vi "UI-copper ring detection.vi"(8 "error in (no error)":errorcluster caption="错误输入（无错误）", 11 "名称或相对路径":string="Template Program") -> (0 "error in (no error) 2":errorcluster caption="错误输入（无错误）")   [LabVIEW 2017]
uses:
  Picture/SaveButtom.ctl
  <vilib>/vision/Measure.llb/Edge Options.ctl
  <vilib>/vision/Measure.llb/Edge Polarity.ctl
  Global System.vi
  <vilib>/Utility/xml.llb/Read From XML File(string).vi
  <vilib>/Utility/xml.llb/Write to XML File(string).vi
panel:
  in  "获取ROI(定位)":bool
  in  "采图按钮":bool
  in  "图像实时显示":bool
  in  "获取ROI(铜环)":bool
  out "Histogram (Histogram 1)":u32[][](array[numeric])
  out "添加的路径":path
  in  "刷新":bool
  in  "测试按钮":bool
  in  "保存按钮":bool
  in  "Main":enum32{"主参数", "圆环中心定位", "检测铜环参数 ", "测试效果"}(tab)
  in  "ParamsUI":T1={"IsNorImage"=TRUE, "Exposure Values"=100289, "ImagePath"=path "C:/Users/hedongpo/Desktop/514-hdp/Alignment Assemble System/Test Picture/B/3.bmp"} caption="参数界面" {"Exposure Values" scale=0.0..200000.0}
  in  "ParamsUI 圆环定位":T5={"圆环ROI设定"={"Center X"=1717, "Center Y"=1486, "Inner Radius"=327, "Outer Radius"=1645, "Start Angle"=0.0, "End Angle"=0.0}, "Options (定位)"={"Search  Direction"=0, "Edge Options"={"Edge Polarity"=0, "Kernel Size"=3, "Width"=3, "Minimum Edge Strength"=50.0, "Interpolation Type"=enum."Bilinear Fixed", "Data Processing Method"=enum."Average"}, "Show Search Area"=TRUE, "Show Search Lines"=TRUE, "Show Edges Found"=TRUE, "Show Result"=TRUE, "Search Area Color"=65280, "Search Lines Color"=255, "Edge Locations Color"=16776960, "Result Color"=16711680, "Overlay Group Name"=""}, "Circle Fit Options (定位)"={"Process"=enum."Get First Edge", "Step Size"=10, "Max Pixel Radius"=3}} caption="参数界面" {"Options (定位)"."Search  Direction" items=["Outside to Inside", "Inside to Outside"]; "Options (定位)"."Edge Options"."Edge Polarity" items=["All Edges", "Rising Edges", "Falling Edges"]; "Options (定位)"."Edge Options"."Minimum Edge Strength" format="%.2f"; "Options (定位)"."Edge Options"."Width" step=2; "Options (定位)"."Edge Options"."Kernel Size" step=2; "圆环ROI设定"."End Angle" min=-90.0 max=90.0 step=1.0 format="%.2f"; "圆环ROI设定"."Start Angle" min=-90.0 max=90.0 step=1.0 format="%.2f"; "圆环ROI设定"."Center X" scale=0.0..1024.0}
  in  "ParamsUI 内圆":cluster{"圆环ROI设定":T2, "黑像素个数判定阀值":dbl}={"圆环ROI设定"={"Center X"=1717, "Center Y"=1486, "Inner Radius"=327, "Outer Radius"=1645, "Start Angle"=0.0, "End Angle"=0.0}, "黑像素个数判定阀值"=0.0} caption="参数界面" {"圆环ROI设定"."End Angle" min=-90.0 max=90.0 step=1.0 format="%.2f"; "圆环ROI设定"."Start Angle" min=-90.0 max=90.0 step=1.0 format="%.2f"; "圆环ROI设定"."Center X" scale=0.0..1024.0}
  out "像素白个数":dbl
  out "像素黑个数":dbl
  out "原始图像":T6(plugin-control)
  out "Histogram 图标":u32[][](graph)
  out "路径输出":path
  in  "Vision Paramter Save Buttom":T7
  out "system time":string
  in  "取消按钮":bool
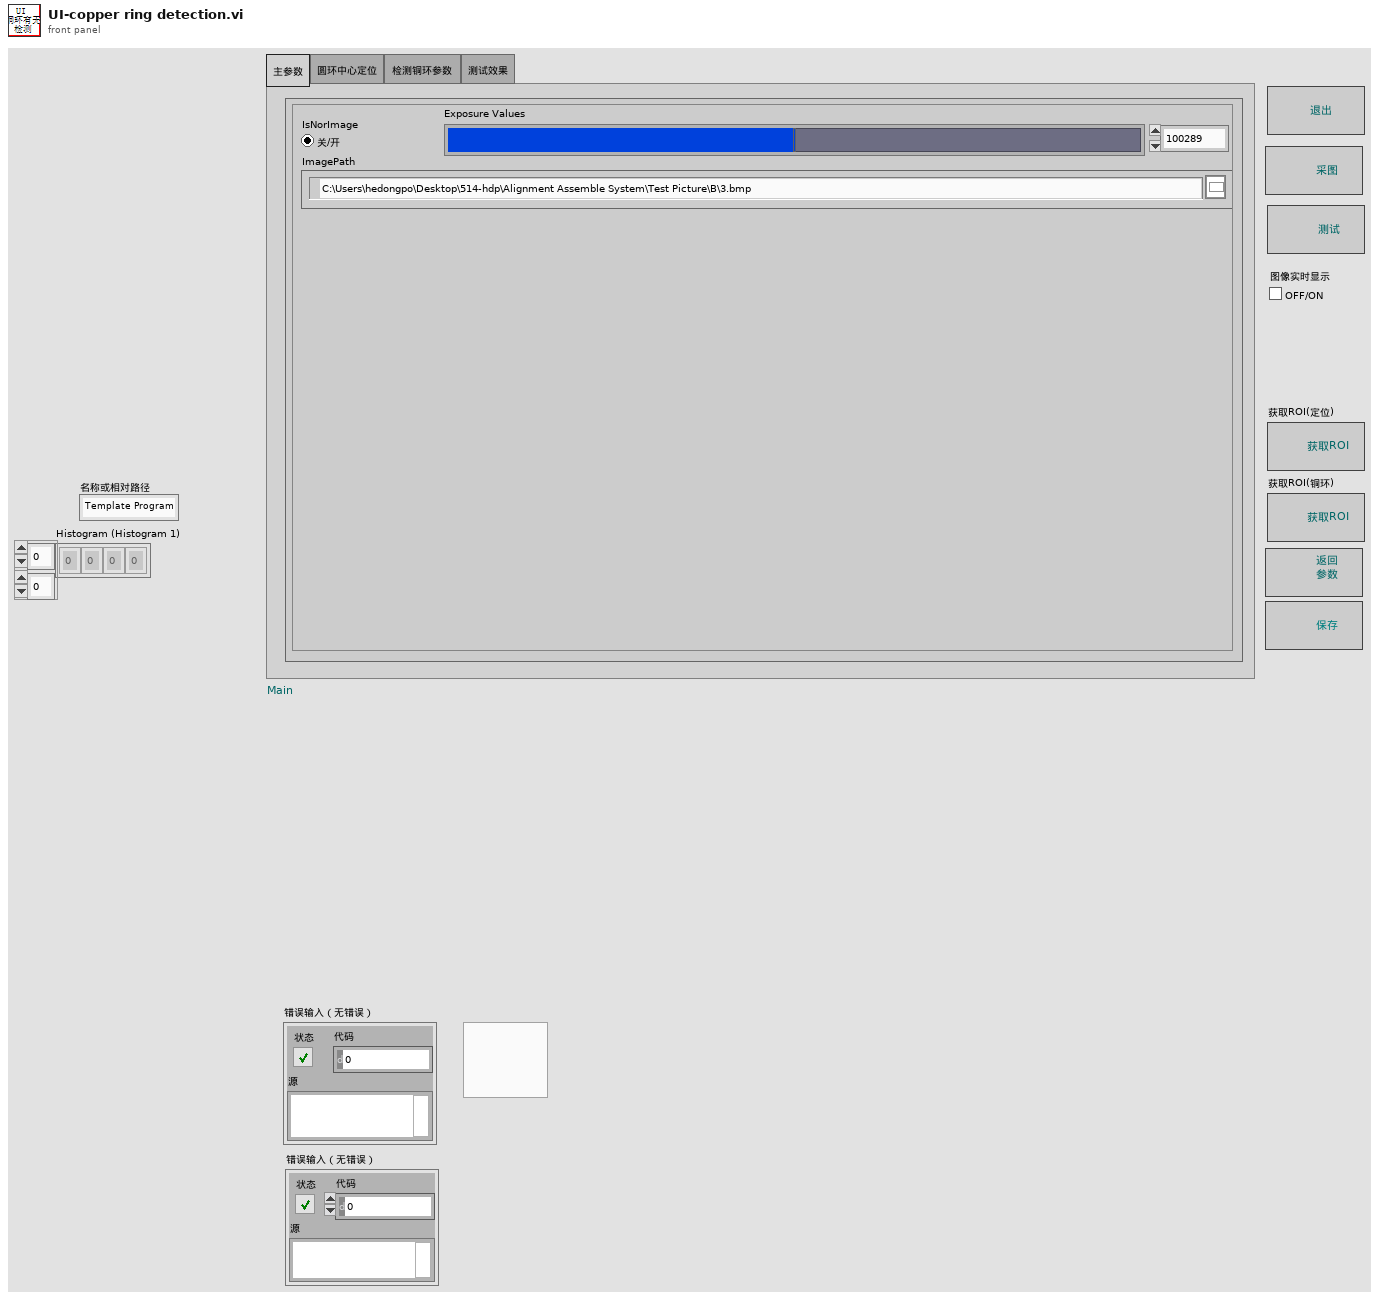
[diagram p1: front panel]
types:
  T1 = cluster{"IsNorImage":bool, "Exposure Values":u32, "ImagePath":path}
  T2 = typedef "IMAQ Circle" = cluster{"Center X":i32, "Center Y":i32, "Inner Radius":i32, "Outer Radius":i32, "Start Angle":dbl, "End Angle":dbl}
  T3 = typedef "Edge Options.ctl" = cluster{"Edge Polarity":T4, "Kernel Size":u32, "Width":u32, "Minimum Edge Strength":sgl, "Interpolation Type":enum32{"Zero Order", "Bilinear", "Quadratic", "Cubic", "Bilinear Fixed"}, "Data Processing Method":enum32{"Average", "Median"}}
  T4 = typedef "Edge Polarity.ctl" = u32
  T5 = cluster{"圆环ROI设定":T2, "Options (定位)":cluster{"Search  Direction":u32, "Edge Options":T3, "Show Search Area":bool, "Show Search Lines":bool, "Show Edges Found":bool, "Show Result":bool, "Search Area Color":u32, "Search Lines Color":u32, "Edge Locations Color":u32, "Result Color":u32, "Overlay Group Name":string}, "Circle Fit Options (定位)":cluster{"Process":enum16{"Get First Edge", "Get First + Last Edge", "Get All Edges", "Get Best Edge"}, "Step Size":i32, "Max Pixel Radius":i32}}
  T6 = typedef "IMAQ Image.ctl" = refnum<image>
  T7 = typedef "SaveButtom.ctl" = bool
  T8 = cluster{"扇区个数":string, "Fitted Circle (Find Circular Edge 1)":cluster{"Center (Pixels)":cluster{"X":sgl, "Y":sgl}, "Radius (Pixels)":dbl, "Center (Real-World)":cluster{"X":sgl, "Y":sgl}, "Radius (Real-World)":dbl, "Roundness (Real-World)":dbl, "Average Strength":dbl, "Average SNR (dB)":dbl}, "Range (Threshold 1)":cluster{"Lower value":sgl, "Upper value":sgl}, "Process (Edge Detector 1)":enum16{"Get First Edge", "Get First + Last Edge", "Get All Edges", "Get Best Edge"}, "Edge Options (Edge Detector 1)":cluster{"Edge Polarity":u32, "Kernel Size":u32, "Width":u32, "Minimum Edge Strength":sgl, "Interpolation Type":enum32{"Zero Order", "Bilinear", "Quadratic", "Cubic", "Bilinear Fixed"}, "Data Processing Method":enum32{"Average", "Median"}}}
  T9 = cluster{"index":i32, "this vi":refnum<vi>, "error out":errorcluster}
  T10 = cluster{"master data":string, "priority":u16, "secondary data":string[]}
  T11 = cluster{"case name":string[], "queue array":refnum<queue>[]}
  T12 = cluster{"Search  Direction":u32, "Edge Options":T3, "Show Search Area":bool, "Show Search Lines":bool, "Show Edges Found":bool, "Show Result":bool, "Search Area Color":u32, "Search Lines Color":u32, "Edge Locations Color":u32, "Result Color":u32, "Overlay Group Name":string}
  T13 = cluster{"Process":enum16{"Get First Edge", "Get First + Last Edge", "Get All Edges", "Get Best Edge"}, "Step Size":i32, "Max Pixel Radius":i32}
  T14 = typedef "ROI Descriptor" = cluster{"Global Rectangle":i32[], "Contours":cluster{"ID":enum32{"External", "Internal"}, "Type":u32, "Coordinates":i32[]}[]}
  T15 = cluster{"Center (Pixels)":cluster{"X":sgl, "Y":sgl}, "Radius (Pixels)":dbl, "Center (Real-World)":cluster{"X":sgl, "Y":sgl}, "Radius (Real-World)":dbl, "Roundness (Real-World)":dbl, "Average Strength":dbl, "Average SNR (dB)":dbl}
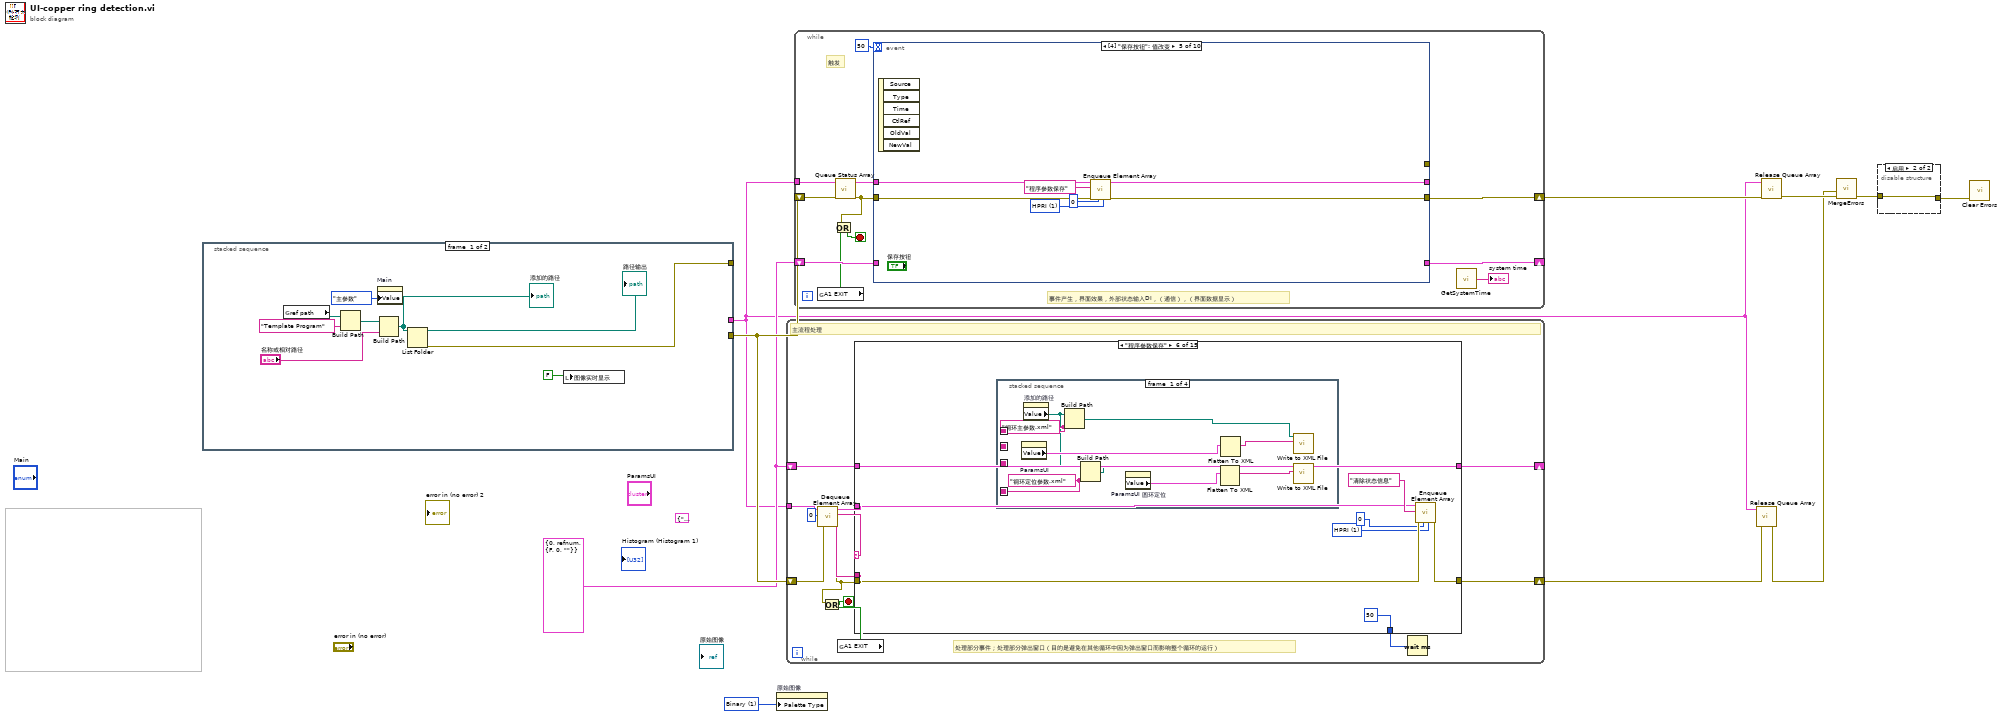
[diagram p0: block diagram]
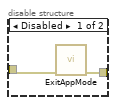
[diagram p2: hidden frame]
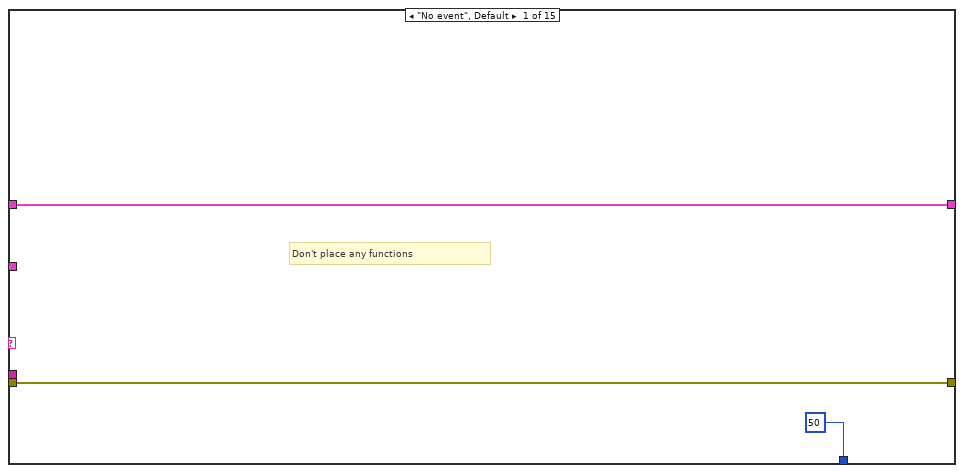
[diagram p3: hidden frame]
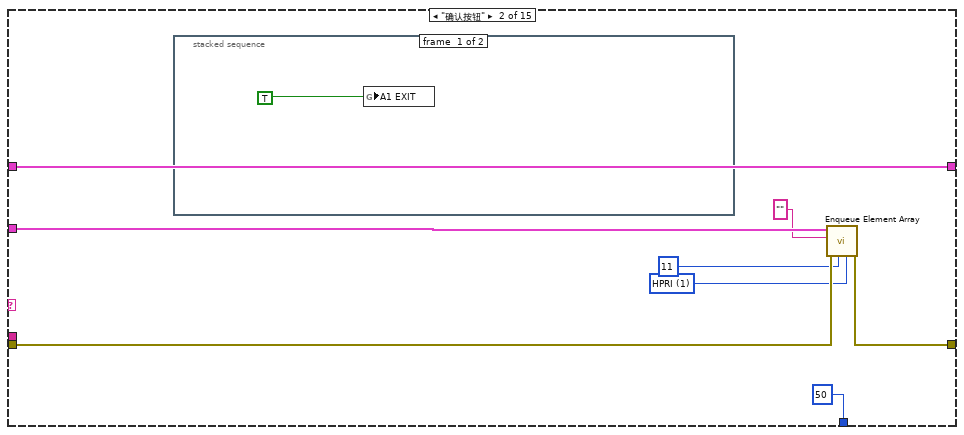
[diagram p4: hidden frame]
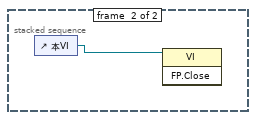
[diagram p5: hidden frame]
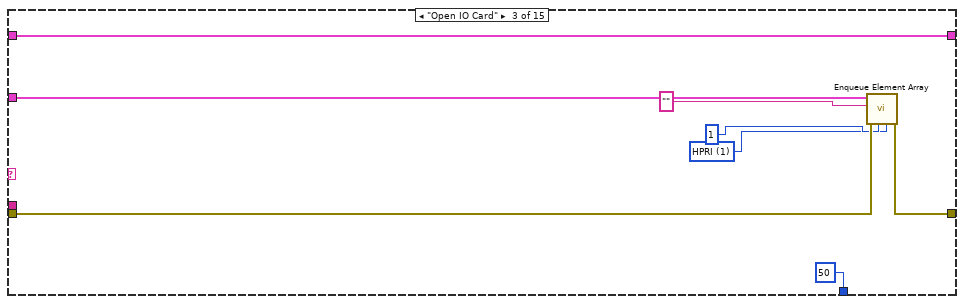
[diagram p6: hidden frame]
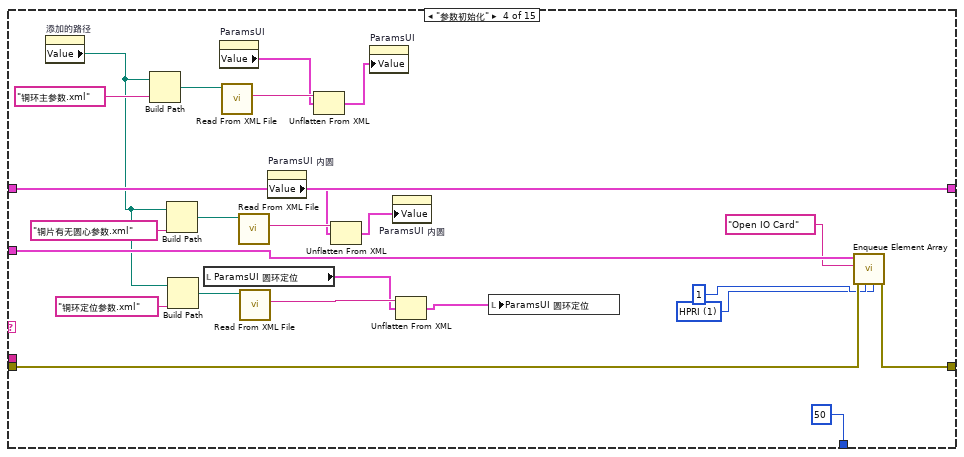
[diagram p7: hidden frame]
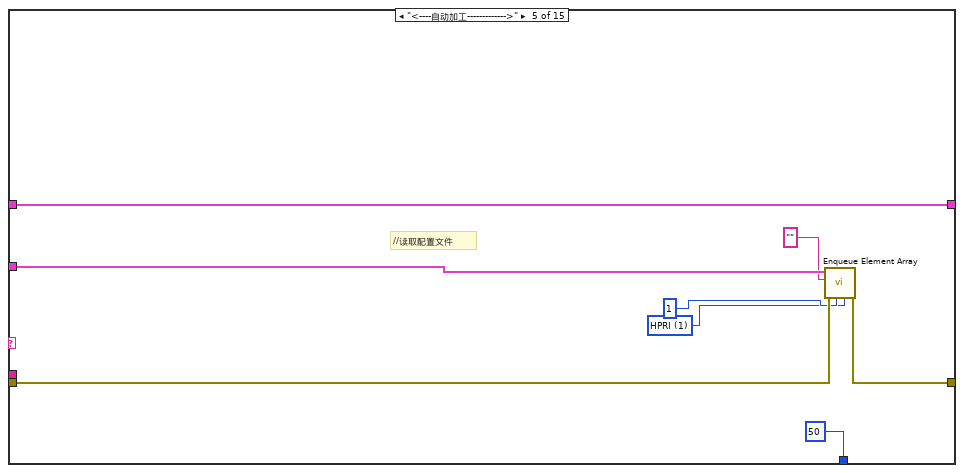
[diagram p8: hidden frame]
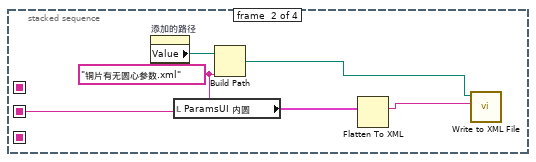
[diagram p9: hidden frame]
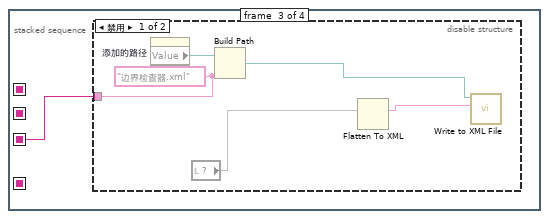
[diagram p10: hidden frame]
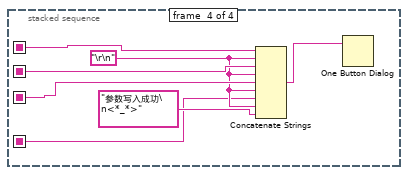
[diagram p12: hidden frame]
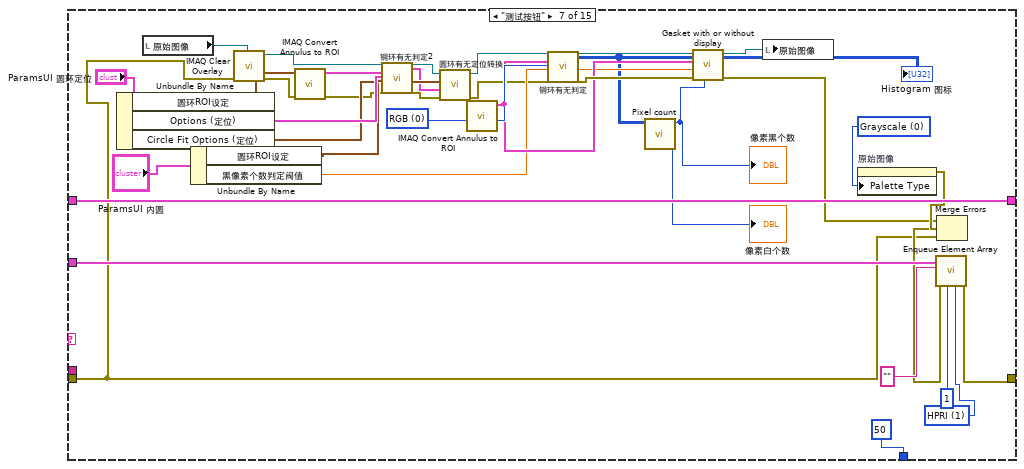
[diagram p13: hidden frame]
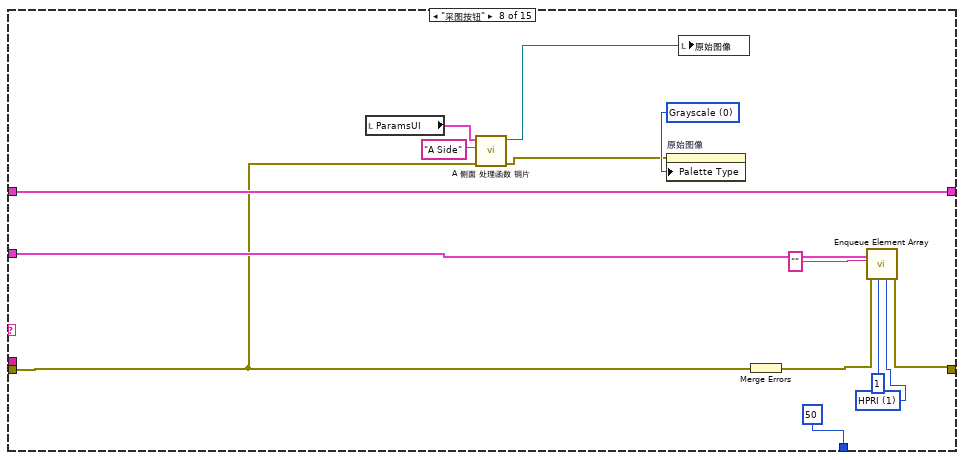
[diagram p14: hidden frame]
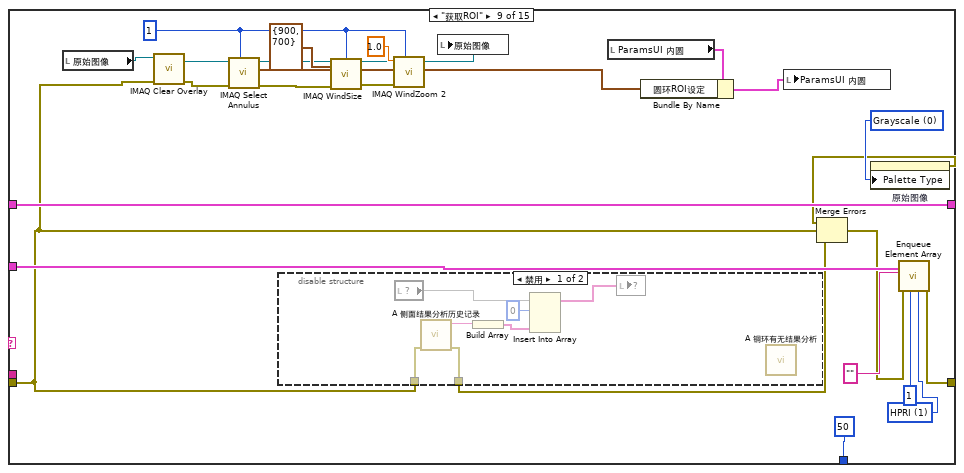
[diagram p15: hidden frame]
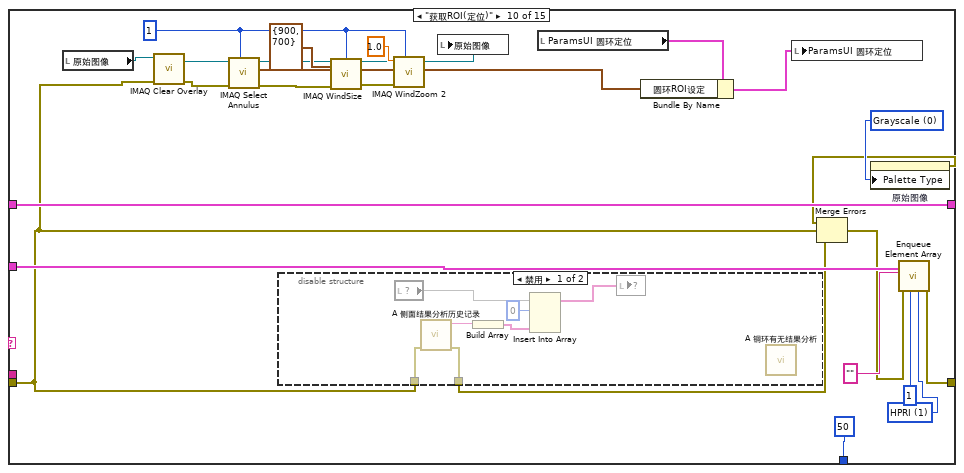
[diagram p17: hidden frame]
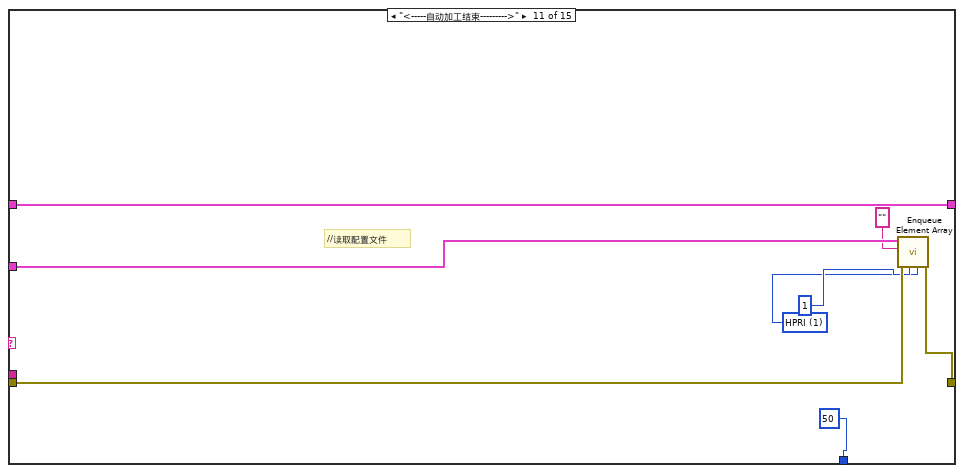
[diagram p19: hidden frame]
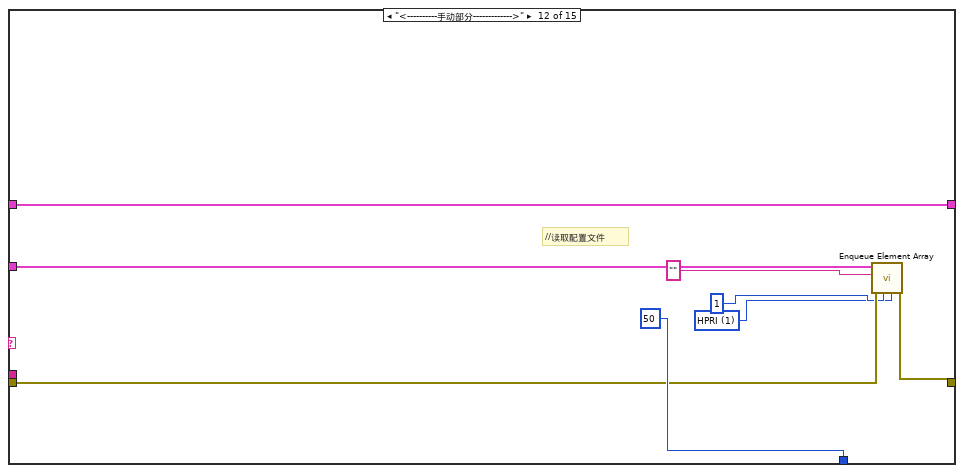
[diagram p20: hidden frame]
diagram:
  (unwired) T8 {"扇区个数"="1", "Fitted Circle (Find Circular Edge 1)"={"Center (Pixels)"={"X"=1736.0, "Y"=1501.0}, "Radius (Pixels)"=1442.0, "Center (Real-World)"={"X"=1736.0, "Y"=1501.0}, "Radius (Real-World)"=1442.0, "Roundness (Real-World)"=0.0, "Average Strength"=0.0, "Average SNR (dB)"=0.0}, "Range (Threshold 1)"={"Lower value"=65.0, "Upper value"=255.0}, "Process (Edge Detector 1)"=enum."Get All Edges", "Edge Options (Edge Detector 1)"={"Edge Polarity"=0, "Kernel Size"=9, "Width"=5, "Minimum Edge Strength"=27.0, "Interpolation Type"=enum."Bilinear", "Data Processing Method"=enum."Average"}} ("边界检查器参数")
  w1 = u32 1 items=["Grayscale", "Binary", "Gradient", "Rainbow", "Temperature", "User Defined", "Binary 16 Bit", "Gradient 16 Bit", "Rainbow 16 Bit", "Temperature 16 Bit", "User Defined 16 Bit"] ("Palette:Palette Type")
  w5 = T9 {"index"=0, "this vi"=refnum, "error out"={"status"=FALSE, "code"=0, "source"=""}} ("parameter buffer")
  n1 = stacked-sequence {
    tunnel: [w17 _] -> _
    tunnel: [_ w21] -> w6
    tunnel: [_ w20] -> w2
    frame #0 {
      n2 = global read "Global System.vi" "ref path"() -> (w15:path)
      n3 = Build Path(base path=w15, name or relative path="Template Program" ("名称或相对路径")) -> (appended path=w13:path)
      n4 = property on="Main" class="TabCtl (严格)"("Value"=enum32{"主参数", "圆环中心定位", "检测铜环参数 ", "测试效果"}."主参数" ("Main")) -> ()  [unwired: 2 in, 2 out]
      n5 = Build Path(base path=w13, name or relative path="名称或相对路径") -> (appended path=w19:path)
      "添加的路径" <- w19
      n6 = List Folder(path=w19) -> (path out=→"路径输出":path, error out=w17:errorcluster)  [unwired: 3 in, 2 out]
      n7 = local write "图像实时显示"(FALSE ("图像实时显示")) -> ()
    }
    frame #1 {
      w29 = string[] ["comm queue1", "data queue 11", "data queue 12", "data queue 13", "data queue 14"]  # queue name
      w30 = 4  # queue num
      w31 = T10 {"master data"="", "priority"=0, "secondary data"=[]}  # element data type
      n8 = call "Obtain Queue Array.vi"("queue name"=w29, "element data type"=w31, "queue num"=w30) -> ("error out"=w25:errorcluster, "queue out"=w26:T11)  [unwired: 2 in, 1 out]
      n9 = call "Enqueue Element Array.vi"("queue index"=0, "error in"=w25, "master data"="参数初始化", "queue in"=w26) -> ("error out"=w24:errorcluster, "queue out"=w23:T11)  [unwired: 6 in]
      n10 = disable-structure shown="启用" {
        disable-tunnel: w24 -> [w37 w38]
        disable-tunnel: w23 -> [w36 w39]
        disable-tunnel: "Loading Variable" ("master data") -> [w35 _]
        disable-tunnel: [w33 w38] -> w21
        disable-tunnel: [w32 w39] -> w20
        frame Disabled {
          n11 = call "Enqueue Element Array.vi"("queue index"=12, "error in"=w37, "master data"=w35, "queue in"=w36) -> ("error out"=w33:errorcluster, "queue out"=w32:T11)  [unwired: 6 in]
        }
        frame Enabled {
        }
      }
    }
  }
  n12 = property on="原始图像" class="ImageControl"("Palette Type"=w1) -> ()  [unwired: 2 in, 2 out]
  n13 = while {
    shift-right: [w52] -> w4
    shift-left: w6 -> [w43]
    shift-right: [w49] -> _
    shift-left: w5 -> [w50]
    tunnel: w2 -> [w45]
    stop <- w40 stop-if-true
    # "处理部分事件；处理部分弹出窗口（目的是避免在其他循环中因为弹出窗口而影响整个循环的运行）"
    # "主流程处理"
    n14 = call "Dequeue Element Array.vi"("queue in"=w45, "queue index"=0, "error in"=w43) -> ("queue out"=w48:T11, "master data"=w47:string, "secondary data"=w46:string[], "error out"=w42:errorcluster)  [unwired: 2 in, 1 out]
    n15 = global read "Global System.vi" "A1 EXIT"() -> (w41:bool)
    n16 = Or(x=w42, y=w41) -> (x .or. y?=w40:bool)
    n17 = case shown="\"程序参数保存\"" w47 {
      tunnel: w48 -> [_ w62 w72 w96 w104 w106 w177 w191 w215 w248 w265 w273 w281 w289 w295]
      tunnel: w42 -> [w54 w58 w68 w93 w100 w110 w143 w179 w195 w230 w261 w269 w277 w285 w292]
      tunnel: [w54 w61 w71 w95 w103 w112 w176 w190 w214 w247 w264 w272 w280 w288 w303] -> w52
      tunnel: [50 50 50 50 50 50 50 50 50 50 50 50 50 50 50] -> w51
      tunnel: w50 -> [w55 w59 w69 w90 w101 w107 w172 w186 w210 w243 w262 w270 w278 w286 w301]
      tunnel: [w55 w59 w69 w90 w101 w107 w172 w186 w210 w243 w262 w270 w278 w286 w301] -> w49
      tunnel: w46 -> [_ _ _ _ _ _ _ _ _ _ _ _ _ _ _]
      frame "No event", Default {
        # "Don't place any functions"
      }
      frame "确认按钮" {
        w56 = u16 1 items=["HPRI"=1, "LPRI"=0] ("priority")
        n18 = stacked-sequence {
          frame #0 {
            n19 = global write "Global System.vi" "A1 EXIT"(TRUE ("EXIT")) -> ()
          }
          frame #1 {
            n20 = control-ref of="本VI"() -> (w65:refnum<vi>)
            n21 = invoke class="VI" method="FP.Close"(reference=w65) -> ()  [unwired: 2 in, 3 out]
          }
        }
        n22 = call "Enqueue Element Array.vi"("priority"=w56, "queue index"=11, "error in"=w58, "master data"="" ("Element 1"), "queue in"=w62) -> ("error out"=w61:errorcluster)  [unwired: 5 in, 1 out]
      }
      frame "Open IO Card" {
        w66 = u16 1 items=["HPRI"=1, "LPRI"=0] ("priority")
        n23 = call "Enqueue Element Array.vi"("priority"=w66, "queue index"=1, "error in"=w68, "master data"="" ("Element 1"), "queue in"=w72) -> ("error out"=w71:errorcluster)  [unwired: 5 in, 1 out]
      }
      frame "参数初始化" {
        w91 = u16 1 items=["HPRI"=1, "LPRI"=0] ("priority")
        n24 = property on="添加的路径" class="Path"() -> ("Value"=w76:path)  [unwired: 2 in, 2 out]
        n25 = Build Path(base path=w76, name or relative path="铜环主参数.xml" ("名称或相对路径")) -> (appended path=w88:path)
        n26 = Build Path(base path=w76, name or relative path="铜片有无圆心参数.xml" ("名称或相对路径")) -> (appended path=w83:path)
        n27 = Build Path(base path=w76, name or relative path="铜环定位参数.xml" ("名称或相对路径")) -> (appended path=w78:path)
        n28 = local read "ParamsUI 圆环定位"() -> (w74:T5)
        n29 = property on="ParamsUI" class="Clust (严格)"() -> ("Value"=w86:T1)  [unwired: 2 in, 2 out]
        n30 = call-poly <vilib>:"Read From XML File.vi"("XML File Path"=w88) -> ("XML Elements"=w87:string)  [unwired: 8 in, 2 out]
        n31 = call-poly <vilib>:"Read From XML File.vi"("XML File Path"=w83) -> ("XML Elements"=w84:string)  [unwired: 8 in, 2 out]
        n32 = call-poly <vilib>:"Read From XML File.vi"("XML File Path"=w78) -> ("XML Elements"=w77:string)  [unwired: 8 in, 2 out]
        n33 = property on="ParamsUI 内圆" class="Clust (严格)"() -> ("Value"=w81:cluster{"圆环ROI设定":T2, "黑像素个数判定阀值":dbl})  [unwired: 2 in, 2 out]
        n34 = Unflatten From XML(xml string=w87, type=w86) -> (value=w85:T1)  [unwired: 1 in, 1 out]
        n35 = Unflatten From XML(xml string=w84, type=w81) -> (value=w80:cluster{"圆环ROI设定":T2, "黑像素个数判定阀值":dbl})  [unwired: 1 in, 1 out]
        n36 = property on="ParamsUI" class="Clust (严格)"("Value"=w85) -> ()  [unwired: 2 in, 2 out]
        n37 = property on="ParamsUI 内圆" class="Clust (严格)"("Value"=w80) -> ()  [unwired: 2 in, 2 out]
        n38 = Unflatten From XML(xml string=w77, type=w74) -> (value=w75:T5)  [unwired: 1 in, 1 out]
        n39 = local write "ParamsUI 圆环定位"(w75) -> ()
        n40 = call "Enqueue Element Array.vi"("priority"=w91, "queue index"=1, "error in"=w93, "master data"="Open IO Card" ("Element 1"), "queue in"=w96) -> ("error out"=w95:errorcluster)  [unwired: 5 in, 1 out]
      }
      frame "<----自动加工------------->" {
        w98 = u16 1 items=["HPRI"=1, "LPRI"=0] ("priority")
        # "//读取配置文件"
        n41 = call "Enqueue Element Array.vi"("priority"=w98, "queue index"=1, "error in"=w100, "master data"="" ("Element 1"), "queue in"=w104) -> ("error out"=w103:errorcluster)  [unwired: 5 in, 1 out]
      }
      frame "程序参数保存" {
        w108 = u16 1 items=["HPRI"=1, "LPRI"=0] ("priority")
        n42 = stacked-sequence {
          seq-local: [w119 _ _ _] -> [_ _ _ w139]
          seq-local: [_ w123 _ _] -> [_ _ _ w137]
          seq-local: [_ _ w128 _] -> [_ _ _ w136]
          seq-local: [w114 _ _ _] -> [_ _ _ w134]
          frame #0 {
            w114 = "铜环定位参数.xml" ("名称或相对路径")
            w119 = "铜环主参数.xml" ("名称或相对路径")
            n43 = property on="ParamsUI" class="Clust (严格)"() -> ("Value"=w122:T1)  [unwired: 2 in, 2 out]
            n44 = property on="添加的路径" class="Path"() -> ("Value"=w118:path)  [unwired: 2 in, 2 out]
            n45 = Build Path(base path=w118, name or relative path=w119) -> (appended path=w120:path)
            n46 = Build Path(base path=w118, name or relative path=w114) -> (appended path=w117:path)
            n47 = property on="ParamsUI 圆环定位" class="Clust (严格)"() -> ("Value"=w116:T5)  [unwired: 2 in, 2 out]
            n48 = Flatten To XML(anything=w116) -> (xml string=w115:string)
            n49 = Flatten To XML(anything=w122) -> (xml string=w121:string)
            n50 = call-poly <vilib>:"Write to XML File.vi"("XML Input"=w121, "XML File Path"=w120) -> ()  [unwired: 7 in, 3 out]
            n51 = call-poly <vilib>:"Write to XML File.vi"("XML Input"=w115, "XML File Path"=w117) -> ()  [unwired: 7 in, 3 out]
          }
          frame #1 {
            w123 = "铜片有无圆心参数.xml" ("名称或相对路径")
            n52 = property on="添加的路径" class="Path"() -> ("Value"=w127:path)  [unwired: 2 in, 2 out]
            n53 = local read "ParamsUI 内圆"() -> (w124:cluster{"圆环ROI设定":T2, "黑像素个数判定阀值":dbl})
            n54 = Build Path(base path=w127, name or relative path=w123) -> (appended path=w125:path)
            n55 = Flatten To XML(anything=w124) -> (xml string=w126:string)
            n56 = call-poly <vilib>:"Write to XML File.vi"("XML Input"=w126, "XML File Path"=w125) -> ()  [unwired: 7 in, 3 out]
          }
          frame #2 {
            n57 = disable-structure shown="禁用" {
              disable-tunnel: [w130 _] -> w128
              frame Disabled {
                w130 = "边界检查器.xml" ("名称或相对路径")
                n58 = property on="添加的路径" class="Path"() -> ("Value"=w133:path)  [unwired: 2 in, 2 out]
                n59 = local read item#-1() -> (w129)
                n60 = Build Path(base path=w133, name or relative path=w130) -> (appended path=w131:path)
                n61 = Flatten To XML(anything=w129) -> (xml string=w132:string)
                n62 = call-poly <vilib>:"Write to XML File.vi"("XML Input"=w132, "XML File Path"=w131) -> ()  [unwired: 7 in, 3 out]
              }
              frame Enabled {
              }
            }
          }
          frame #3 {
            w135 = "\r\n"
            n63 = Concatenate Strings(w139, w135, w137, w135, w136, w135, w134, w135, "参数写入成功\n<*_*>" ("消息")) -> (w138:string)
            n64 = One Button Dialog(message=w138) -> ()  [unwired: 1 in, 1 out]
          }
        }
        n65 = call "Enqueue Element Array.vi"("priority"=w108, "queue index"=0, "error in"=w110, "master data"="清除状态信息" ("Element 1"), "queue in"=w106) -> ("error out"=w112:errorcluster)  [unwired: 5 in, 1 out]
      }
      frame "测试按钮" {
        w167 = u16 0 items=["RGB", "HSL", "HSV", "HSI"] ("Color Mode (Histogram 1)")
        w171 = u32 0 items=["Grayscale", "Binary", "Gradient", "Rainbow", "Temperature", "User Defined", "Binary 16 Bit", "Gradient 16 Bit", "Rainbow 16 Bit", "Temperature 16 Bit", "User Defined 16 Bit"] ("Palette:Palette Type")
        w173 = u16 1 items=["HPRI"=1, "LPRI"=0] ("priority")
        n66 = Unbundle By Name("ParamsUI 圆环定位") -> ("圆环ROI设定"=w156:T2, "Options (定位)"=w154:T12, "Circle Fit Options (定位)"=w153:T13)
        n67 = local read "原始图像"() -> (w158:T6)
        n68 = Unbundle By Name("ParamsUI 内圆") -> ("圆环ROI设定"=w152:T2, "黑像素个数判定阀值"=w160:dbl)
        n69 = call "IMAQ Clear Overlay"("error in (no error)"=w143, "Image"=w158) -> ("error out"=w144:errorcluster, "Image Out"=w145:T6)  [unwired: 8 in]
        n70 = call "IMAQ Convert Annulus to ROI"("error in (no error)"=w144, "Annulus"=w156) -> ("error out"=w142:errorcluster, "ROI Descriptor"=w155:T14)  [unwired: 7 in]
        n71 = call "铜环有无判定2"("Image In"=w145, "ROI Descriptor (Find Circular Edge 1)"=w155, "Options (Find Circular Edge 1)"=w154, "Circle Fit Options (Find Circular Edge 1)"=w153, "error in"=w142) -> ("Image Out"=w149:T6, "Fitted Circle (Find Circular Edge 1)"=w150:T15, "error out"=w147:errorcluster)  [unwired: 20 in]
        n72 = call "圆环有无定位转换.vi"("error in (no error)"=w147, "Fitted Circle (定位)"=w150, "圆环ROI设定 in"=w152, "Image in"=w149) -> ("error out"=w146:errorcluster, "圆环ROI设定 out"=w151:T2, "Image out"=w148:T6)  [unwired: 4 in, 1 out]
        n73 = call "IMAQ Convert Annulus to ROI"("Annulus"=w151) -> ("ROI Descriptor"=w162:T14)  [unwired: 8 in, 1 out]
        n74 = call "铜环有无判定"("Image In"=w148, "ROI Descriptor (Histogram 1)"=w162, "Color Mode (Histogram 1)"=w167, "error in"=w146) -> ("Image Out"=w166:T6, "Histogram (Histogram 1)"=w141:u32[][], "error out"=w164:errorcluster)  [unwired: 20 in, 1 out]
        "Histogram 图标" <- w141
        n75 = call "Pixel count.vi"("Histogram 图标"=w141) -> ("像素白个数"=→"像素白个数":u32, "像素黑个数"=w159:u32)  [unwired: 9 in]
        "像素黑个数" <- w159
        n76 = call "Gasket with or without display.vi"("黑像个数"=w159, "error in (no error)"=w164, "黑像素阀值判定个数"=w160, "ROI Descriptor"=w162, "原始图像 IN"=w166) -> ("error out"=w163:errorcluster, "原始图像 OUT"=w165:T6)  [unwired: 3 in, 2 out]
        n77 = local write "原始图像"(w165) -> ()
        n78 = property on="原始图像" class="ImageControl"("Palette Type"=w171) -> (error out=w170:errorcluster)  [unwired: 2 in, 1 out]
        n79 = Merge Errors(w163, w170, w143) -> (w169:errorcluster)
        n80 = call "Enqueue Element Array.vi"("priority"=w173, "queue index"=1, "error in"=w169, "master data"="" ("Element 1"), "queue in"=w177) -> ("error out"=w176:errorcluster)  [unwired: 5 in, 1 out]
      }
      frame "采图按钮" {
        w184 = u32 0 items=["Grayscale", "Binary", "Gradient", "Rainbow", "Temperature", "User Defined", "Binary 16 Bit", "Gradient 16 Bit", "Rainbow 16 Bit", "Temperature 16 Bit", "User Defined 16 Bit"] ("Palette:Palette Type")
        w187 = u16 1 items=["HPRI"=1, "LPRI"=0] ("priority")
        n81 = local read "ParamsUI"() -> (w183:T1)
        n82 = call "A 侧面 处理函数 铜片.vi"("error in (no error)"=w179, "Image Name"="A Side", "ParamsUI"=w183) -> ("error out"=w180:errorcluster, "Image out"=w181:T6)  [unwired: 5 in, 2 out]
        n83 = property on="原始图像" class="ImageControl"(error in=w180, "Palette Type"=w184) -> ()  [unwired: 1 in, 2 out]
        n84 = local write "原始图像"(w181) -> ()
        n85 = Merge Errors(w179) -> (w182:errorcluster)
        n86 = call "Enqueue Element Array.vi"("priority"=w187, "queue index"=1, "error in"=w182, "master data"="" ("Element 1"), "queue in"=w191) -> ("error out"=w190:errorcluster)  [unwired: 5 in, 1 out]
      }
      frame "获取ROI" {
        w203 = 1 ("Window Number (0...15)")
        w209 = u32 0 items=["Grayscale", "Binary", "Gradient", "Rainbow", "Temperature", "User Defined", "Binary 16 Bit", "Gradient 16 Bit", "Rainbow 16 Bit", "Temperature 16 Bit", "User Defined 16 Bit"] ("Palette:Palette Type")
        w211 = u16 1 items=["HPRI"=1, "LPRI"=0] ("priority")
        n87 = local read "原始图像"() -> (w196:T6)
        n88 = call "IMAQ Clear Overlay"("error in (no error)"=w195, "Image"=w196) -> ("error out"=w194:errorcluster, "Image Out"=w193:T6)  [unwired: 8 in]
        n89 = call "IMAQ Select Annulus"("Window Number (0...15)"=w203, "error in (no error)"=w194, "Image In"=w193) -> ("error out"=w205:errorcluster, "Annulus"=w198:T2, "Image Out (duplicate)"=w200:T6)  [unwired: 5 in, 1 out]
        n90 = disable-structure shown="禁用" {
          disable-tunnel: w195 -> [w220 _]
          disable-tunnel: [w219 _] -> w206
          frame Disabled {
            n91 = local read item#-1() -> (w218)
            n92 = call "A 侧面结果分析历史记录.vi"("错误输入（无错误）"=w220) -> ("错误输出"=w219:errorcluster, "F-格式字符串"=w223:string, "Tbl引用句柄"=w221:refnum<vi>)  [unwired: 8 in]
            n93 = Build Array(w223) -> (w222:string[])
            n94 = Insert Into Array(array=w218, index (row)=0 ("索引 (行)"), new element=w222) -> (w217:string[])  [unwired: 1 in]
            n95 = local write item#-1(w217) -> ()
            n96 = call "A 铜环有无结果分析.vi"() -> ("Tbl引用句柄"=w225:refnum<vi>)  [unwired: 11 in]
          }
          frame Enabled {
          }
        }
        n97 = call "IMAQ WindSize"("error in (no error)"=w205, "Width & Height"=cluster{"Width":i32, "Height":i32} {"Width"=900, "Height"=700}, "Window Number"=w203) -> ("error out"=w202:errorcluster)  [unwired: 3 in, 2 out]
        n98 = call "IMAQ WindZoom 2"("Window Number (0...15)"=w203, "error in (no error)"=w202, "Zoom Factor"=sgl 1.0) -> ()  [unwired: 5 in, 4 out]
        n99 = local write "原始图像"(w200) -> ()
        n100 = local read "ParamsUI 内圆"() -> (w199:cluster{"圆环ROI设定":T2, "黑像素个数判定阀值":dbl})
        n101 = Bundle By Name(cluster=w199, "圆环ROI设定"=w198) -> (w197:cluster{"圆环ROI设定":T2, "黑像素个数判定阀值":dbl})
        n102 = local write "ParamsUI 内圆"(w197) -> ()
        n103 = property on="原始图像" class="ImageControl"("Palette Type"=w209) -> (error out=w208:errorcluster)  [unwired: 2 in, 1 out]
        n104 = Merge Errors(w208, w195, w206) -> (w207:errorcluster)
        n105 = call "Enqueue Element Array.vi"("priority"=w211, "queue index"=1, "error in"=w207, "master data"="" ("Element 1"), "queue in"=w215) -> ("error out"=w214:errorcluster)  [unwired: 5 in, 1 out]
      }
      frame "获取ROI(定位)" {
        w236 = 1 ("Window Number (0...15)")
        w242 = u32 0 items=["Grayscale", "Binary", "Gradient", "Rainbow", "Temperature", "User Defined", "Binary 16 Bit", "Gradient 16 Bit", "Rainbow 16 Bit", "Temperature 16 Bit", "User Defined 16 Bit"] ("Palette:Palette Type")
        w244 = u16 1 items=["HPRI"=1, "LPRI"=0] ("priority")
        n106 = local read "原始图像"() -> (w231:T6)
        n107 = call "IMAQ Clear Overlay"("error in (no error)"=w230, "Image"=w231) -> ("error out"=w229:errorcluster, "Image Out"=w228:T6)  [unwired: 8 in]
        n108 = call "IMAQ Select Annulus"("Window Number (0...15)"=w236, "error in (no error)"=w229, "Image In"=w228) -> ("error out"=w238:errorcluster, "Annulus"=w232:T2, "Image Out (duplicate)"=w233:T6)  [unwired: 5 in, 1 out]
        n109 = disable-structure shown="禁用" {
          disable-tunnel: w230 -> [w253 _]
          disable-tunnel: [w252 _] -> w239
          frame Disabled {
            n110 = local read item#-1() -> (w251)
            n111 = call "A 侧面结果分析历史记录.vi"("错误输入（无错误）"=w253) -> ("错误输出"=w252:errorcluster, "F-格式字符串"=w256:string, "Tbl引用句柄"=w254:refnum<vi>)  [unwired: 8 in]
            n112 = Build Array(w256) -> (w255:string[])
            n113 = Insert Into Array(array=w251, index (row)=0 ("索引 (行)"), new element=w255) -> (w250:string[])  [unwired: 1 in]
            n114 = local write item#-1(w250) -> ()
            n115 = call "A 铜环有无结果分析.vi"() -> ("Tbl引用句柄"=w258:refnum<vi>)  [unwired: 11 in]
          }
          frame Enabled {
          }
        }
        n116 = call "IMAQ WindSize"("error in (no error)"=w238, "Width & Height"=cluster{"Width":i32, "Height":i32} {"Width"=900, "Height"=700}, "Window Number"=w236) -> ("error out"=w235:errorcluster)  [unwired: 3 in, 2 out]
        n117 = call "IMAQ WindZoom 2"("Window Number (0...15)"=w236, "error in (no error)"=w235, "Zoom Factor"=sgl 1.0) -> ()  [unwired: 5 in, 4 out]
        n118 = local write "原始图像"(w233) -> ()
        n119 = local read "ParamsUI 圆环定位"() -> (w227:T5)
        n120 = Bundle By Name(cluster=w227, "圆环ROI设定"=w232) -> (w226:T5)
        n121 = local write "ParamsUI 圆环定位"(w226) -> ()
        n122 = property on="原始图像" class="ImageControl"("Palette Type"=w242) -> (error out=w241:errorcluster)  [unwired: 2 in, 1 out]
        n123 = Merge Errors(w241, w230, w239) -> (w240:errorcluster)
        n124 = call "Enqueue Element Array.vi"("priority"=w244, "queue index"=1, "error in"=w240, "master data"="" ("Element 1"), "queue in"=w248) -> ("error out"=w247:errorcluster)  [unwired: 5 in, 1 out]
      }
      frame "<-----自动加工结束--------->" {
        w259 = u16 1 items=["HPRI"=1, "LPRI"=0] ("priority")
        # "//读取配置文件"
        n125 = call "Enqueue Element Array.vi"("priority"=w259, "queue index"=1, "error in"=w261, "master data"="" ("Element 1"), "queue in"=w265) -> ("error out"=w264:errorcluster)  [unwired: 5 in, 1 out]
      }
      frame "<----------手动部分------------->" {
        w267 = u16 1 items=["HPRI"=1, "LPRI"=0] ("priority")
        # "//读取配置文件"
        n126 = call "Enqueue Element Array.vi"("priority"=w267, "queue index"=1, "error in"=w269, "master data"="" ("Element 1"), "queue in"=w273) -> ("error out"=w272:errorcluster)  [unwired: 5 in, 1 out]
      }
      frame "参数设置保存" {
        w275 = u16 1 items=["HPRI"=1, "LPRI"=0] ("priority")
        n127 = call "Enqueue Element Array.vi"("priority"=w275, "queue index"=1, "error in"=w277, "master data"="" ("Element 1"), "queue in"=w281) -> ("error out"=w280:errorcluster)  [unwired: 5 in, 1 out]
      }
      frame "<--------------手动结束---------------->" {
        w283 = u16 1 items=["HPRI"=1, "LPRI"=0] ("priority")
        # "//读取配置文件"
        n128 = call "Enqueue Element Array.vi"("priority"=w283, "queue index"=1, "error in"=w285, "master data"="" ("Element 1"), "queue in"=w289) -> ("error out"=w288:errorcluster)  [unwired: 5 in, 1 out]
      }
      frame "*Emergency alarm" {
        w298 = u16 1 items=["HPRI"=1, "LPRI"=0] ("priority")
        w299 = u16 1 items=["HPRI"=1, "LPRI"=0] ("priority")
        # "发出处理急停信号的命令"
        # "发出处理急停信号的命令"
        n129 = call "Enqueue Element Array.vi"("priority"=w298, "queue index"=0, "error in"=w292, "master data"="" ("Element 1"), "queue in"=w295) -> ("error out"=w293:errorcluster, "queue out"=w294:T11)  [unwired: 5 in]
        n130 = call "SetTestInfoIndex.vi"("test info index"=13) -> ()
        n131 = call "Enqueue Element Array.vi"("priority"=w299, "queue index"=1, "error in"=w293, "master data"="" ("Element 1"), "queue in"=w294) -> ("error out"=w303:errorcluster)  [unwired: 5 in, 1 out]
      }
    }
    n132 = Wait (ms)(milliseconds to wait=w51) -> ()  [unwired: 1 out]
  }
  n133 = while {
    shift-right: [w308] -> w7
    shift-left: w6 -> [w312]
    shift-right: [w310] -> _
    shift-left: w5 -> [w311]
    tunnel: w2 -> [w314]
    stop <- w305 stop-if-true
    # "触发"
    # "事件产生，界面效果，外部状态输入DI，（通信），（界面数据显示）"
    n134 = global read "Global System.vi" "A1 EXIT"() -> (w306:bool)
    n135 = call "Queue Status Array.vi"("error in (no error)"=w312, "queue in"=w314) -> ("error out"=w307:errorcluster, "queue out"=w309:T11)  [unwired: 4 in]
    n136 = Or(x=w307, y=w306) -> (x .or. y?=w305:bool)
    n137 = event shown="[4] \"保存按钮\": 值改变" {
      selector: _ -> [_ _ _ _ _ _ _ _ _ _]
      dyn-events: _ -> [_ _ _ _ _ _ _ _ _ _]
      timeout: 50 -> [_ _ _ _ _ _ _ _ _ _]
      tunnel: w311 -> [w320 w334 _ _ _ _ _ _ _ _]
      tunnel: [w320 w334 _ _ _ _ _ _ _ _] -> w310
      tunnel: [errorcluster {"status"=FALSE, "code"=0, "source"=""} ("error out") _ _ _ _ _ _ _ _ _] -> _
      tunnel: w309 -> [w318 w333 w339 w346 w353 w361 w369 w377 w385 w393]
      tunnel: w307 -> [w316 w332 w338 w345 w352 w360 w368 w376 w384 w392]
      tunnel: [w316 w331 w336 w343 w350 w358 w366 w374 w382 w390] -> w308
      tunnel: [w318 w330 w337 w344 w351 w359 w367 w375 w383 w391] -> _
      event Timeout {
        # "不要在事件结构里面放入\"弹出窗口\"这样的VI保证该循环畅通无阻。"
        n138 = event-data() -> ()  [unwired: 1 in, 1 out]
        n139 = case shown="真" "图像实时显示" {
          tunnel: w316 -> [_ w321]
          frame False {
          }
          frame True {
            w323 = u32 0 items=["Grayscale", "Binary", "Gradient", "Rainbow", "Temperature", "User Defined", "Binary 16 Bit", "Gradient 16 Bit", "Rainbow 16 Bit", "Temperature 16 Bit", "User Defined 16 Bit"] ("Palette:Palette Type")
            n140 = local read "ParamsUI"() -> (w326:T1)
            n141 = call "Get aperture images CCD2.vi"("error in (no error)"=w321, "Image Name"="A Side", "ParamsUI"=w326) -> ("error out"=w322:errorcluster, "Image out"=w324:T6)  [unwired: 5 in, 2 out]
            n142 = property on="原始图像" class="ImageControl"(error in=w322, "Palette Type"=w323) -> ()  [unwired: 1 in, 2 out]
            n143 = local write "原始图像"(w324) -> ()
          }
        }
      }
      event Panel Close? {
        w328 = u16 1 items=["HPRI"=1, "LPRI"=0] ("priority")
        n144 = event-data() -> ()  [unwired: 1 in, 4 out]
        n145 = call "Enqueue Element Array.vi"("priority"=w328, "queue index"=0, "error in"=w332, "master data"="*Exit application", "queue in"=w333) -> ("error out"=w331:errorcluster, "queue out"=w330:T11)  [unwired: 5 in]
        n146 = event-data("Discard?"=TRUE) -> ()  [unwired: 1 in, 1 out]
      }
      event Value Change {
        w341 = u16 1 items=["HPRI"=1, "LPRI"=0] ("priority")
        n147 = event-data() -> ()  [unwired: 1 in, 6 out]
        n148 = call "Enqueue Element Array.vi"("priority"=w341, "queue index"=0, "error in"=w338, "master data"="Vision Paramter Save", "queue in"=w339) -> ("error out"=w336:errorcluster, "queue out"=w337:T11)  [unwired: 5 in]
      }
      event "取消按钮": Value Change {
        w348 = u16 1 items=["HPRI"=1, "LPRI"=0] ("priority")
        n149 = event-data() -> ()  [unwired: 1 in, 6 out]
        n150 = call "Enqueue Element Array.vi"("priority"=w348, "queue index"=0, "error in"=w345, "master data"="确认按钮", "queue in"=w346) -> ("error out"=w343:errorcluster, "queue out"=w344:T11)  [unwired: 5 in]
      }
      event "保存按钮": Value Change {
        w355 = u16 1 items=["HPRI"=1, "LPRI"=0] ("priority")
        n151 = event-data() -> ()  [unwired: 1 in, 6 out]
        n152 = call "Enqueue Element Array.vi"("priority"=w355, "queue index"=0, "error in"=w352, "master data"="程序参数保存", "queue in"=w353) -> ("error out"=w350:errorcluster, "queue out"=w351:T11)  [unwired: 5 in]
      }
      event "测试按钮": Value Change {
        w363 = u16 1 items=["HPRI"=1, "LPRI"=0] ("priority")
        n153 = event-data() -> ()  [unwired: 1 in, 6 out]
        n154 = property on="Main" class="TabCtl (严格)"("Value"=enum32{"主参数", "圆环中心定位", "检测铜环参数 ", "测试效果"}."测试效果" ("Main")) -> ()  [unwired: 2 in, 2 out]
        n155 = call "Enqueue Element Array.vi"("priority"=w363, "queue index"=0, "error in"=w360, "master data"="测试按钮", "queue in"=w361) -> ("error out"=w358:errorcluster, "queue out"=w359:T11)  [unwired: 5 in]
      }
      event "采图按钮": Value Change {
        w371 = u16 1 items=["HPRI"=1, "LPRI"=0] ("priority")
        n156 = event-data() -> ()  [unwired: 1 in, 6 out]
        n157 = property on="Main" class="TabCtl (严格)"("Value"=enum32{"主参数", "圆环中心定位", "检测铜环参数 ", "测试效果"}."测试效果" ("Main")) -> ()  [unwired: 2 in, 2 out]
        n158 = call "Enqueue Element Array.vi"("priority"=w371, "queue index"=0, "error in"=w368, "master data"="采图按钮", "queue in"=w369) -> ("error out"=w366:errorcluster, "queue out"=w367:T11)  [unwired: 5 in]
      }
      event "获取ROI(铜环)": Value Change {
        w379 = u16 1 items=["HPRI"=1, "LPRI"=0] ("priority")
        n159 = event-data() -> ()  [unwired: 1 in, 6 out]
        n160 = property on="Main" class="TabCtl (严格)"("Value"=enum32{"主参数", "圆环中心定位", "检测铜环参数 ", "测试效果"}."测试效果" ("Main")) -> ()  [unwired: 2 in, 2 out]
        n161 = call "Enqueue Element Array.vi"("priority"=w379, "queue index"=0, "error in"=w376, "master data"="获取ROI", "queue in"=w377) -> ("error out"=w374:errorcluster, "queue out"=w375:T11)  [unwired: 5 in]
      }
      event "获取ROI(定位)": Value Change {
        w387 = u16 1 items=["HPRI"=1, "LPRI"=0] ("priority")
        n162 = event-data() -> ()  [unwired: 1 in, 6 out]
        n163 = property on="Main" class="TabCtl (严格)"("Value"=enum32{"主参数", "圆环中心定位", "检测铜环参数 ", "测试效果"}."测试效果" ("Main")) -> ()  [unwired: 2 in, 2 out]
        n164 = call "Enqueue Element Array.vi"("priority"=w387, "queue index"=0, "error in"=w384, "master data"="获取ROI(定位)", "queue in"=w385) -> ("error out"=w382:errorcluster, "queue out"=w383:T11)  [unwired: 5 in]
      }
      event "刷新": Value Change {
        n165 = event-data() -> ()  [unwired: 1 in, 6 out]
        n166 = disable-structure shown="禁用" {
          disable-tunnel: w393 -> [w397 _]
          disable-tunnel: w392 -> [w396 _]
          disable-tunnel: [w395 _] -> w391
          disable-tunnel: [w394 _] -> w390
          frame Disabled {
            w399 = u16 1 items=["HPRI"=1, "LPRI"=0] ("priority")
            # "刷新"
            n167 = call "Enqueue Element Array.vi"("priority"=w399, "queue index"=0, "error in"=w396, "master data"="刷新", "queue in"=w397) -> ("error out"=w394:errorcluster, "queue out"=w395:T11)  [unwired: 5 in]
          }
          frame Enabled {
          }
        }
        n168 = property on="Main" class="TabCtl (严格)"("Value"=enum32{"主参数", "圆环中心定位", "检测铜环参数 ", "测试效果"}."检测铜环参数 " ("Main")) -> ()  [unwired: 2 in, 2 out]
      }
    }
    n169 = call "GetSystemTime.vi"() -> ("date/time string"=→"system time":string)  [unwired: 7 in]
  }
  n170 = call "Release Queue Array.vi"("error in"=w4, "queue in"=w2) -> ("error out"=w3:errorcluster)  [unwired: 2 in, 3 out]
  n171 = call "Release Queue Array.vi"("error in"=w7, "queue in"=w2) -> ("error out"=w10:errorcluster)  [unwired: 2 in, 3 out]
  n172 = call "MergeErrors.vi"("error in 3 (no error)"=w3, "error in 4 (no error)"=w10) -> ("error out"=w9:errorcluster)  [unwired: 6 in]
  n173 = disable-structure shown="启用" {
    disable-tunnel: w9 -> [w402 w403]
    disable-tunnel: [w401 w403] -> w8
    frame Disabled {
      n174 = call "ExitAppMode.vi"("error in (no error)"=w402) -> ("error out"=w401:errorcluster)  [unwired: 10 in]
    }
    frame Enabled {
    }
  }
  n175 = call <vilib>:"Clear Errors.vi"("error in (no error)"=w8) -> ()  [unwired: 5 in, 2 out]
